vi "Close.vi"(0 "error handler in":refnum<class "TLB` Error Handler.lvclass">, 11 "error in":errorcluster) -> (15 "error out":errorcluster)   [LabVIEW 2023, in "TLB` InstStu GPlugin Template.lvlib" / "TLB` Error Handler.lvclass"]
doc: "Close error handler resources.\n\n<B>Input Parameters</B>\n\n<B>error handler in</B> identifies your session. <B>Error Handler in</B> is obtained from the Open.vi of this class.\n\n<B>error in</B> describes error conditions that occur before this node runs. This input provides standard error in functionality.\n\n<B>Output Parameters</B>\n\n<B>error out</B> contains error information. This output provides standard error out functionality."
uses:
  TLB` Error Handler.lvclass
  TLB` Error Handler.lvclass/TLB` Error Handler.ctl
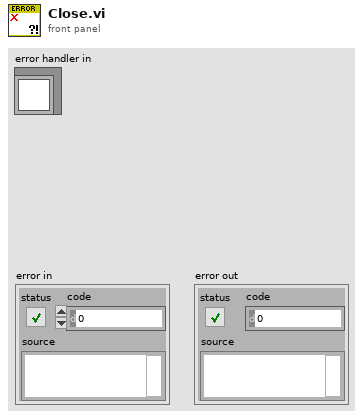
[diagram p1: front panel]
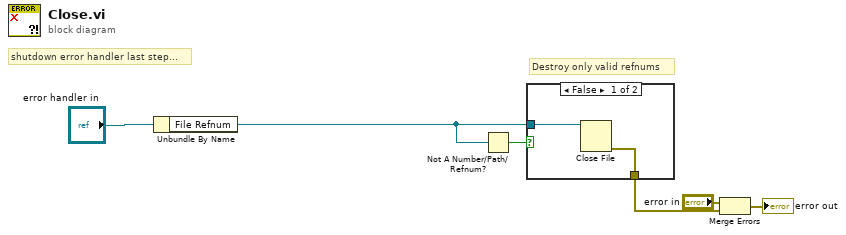
[diagram p0: block diagram]
diagram:
  # "shutdown error handler last step..."
  # "Destroy only valid refnums"
  n1 = Unbundle By Name("error handler in") -> ("File Refnum"=w5:refnum<file>)
  n2 = Not A Number/Path/Refnum?(number/path/refnum=w5) -> (NaN/Path/Refnum?=w6:bool)
  n3 = case shown="False" w6 {
    tunnel: w5 -> [w8 _]
    tunnel: [w7 _] -> w2
    frame False {
      n4 = Close File(refnum=w8) -> (error out=w7:errorcluster)  [unwired: 1 in, 1 out]
    }
    frame True {
    }
  }
  n5 = Merge Errors("error in", w2) -> (→"error out":errorcluster)
